vi "New Worker Name UI.vi"(11 "Starting Name":string) -> (0 "New Project?":bool, 1 "Add to Project":refnum<vi>, 2 "Cancelled?":bool, 3 "New Name":string)   [LabVIEW 2020, in "FlexBlocks.lvlib"]
uses:
  FlexBlocks.lvlib
panel:
  in  "Project":string(combo)
  in  "Add To Project":bool
  in  "Cancel":bool
  in  "OK":bool
  # "Enter the name of the new Worker to create:"
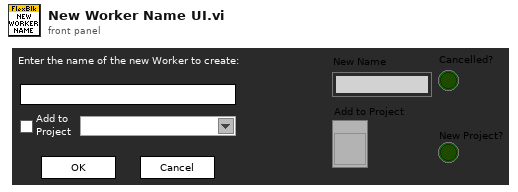
[diagram p1: front panel]
types:
  T1 = typedef "FlexBlocks.lvlib/Paths.ctl" = cluster{"FlexBlocks":path, "Workers Root":path, "Specialized Editors":path, "Worker Template":path, "Editor Template":path, "Express Template":path}
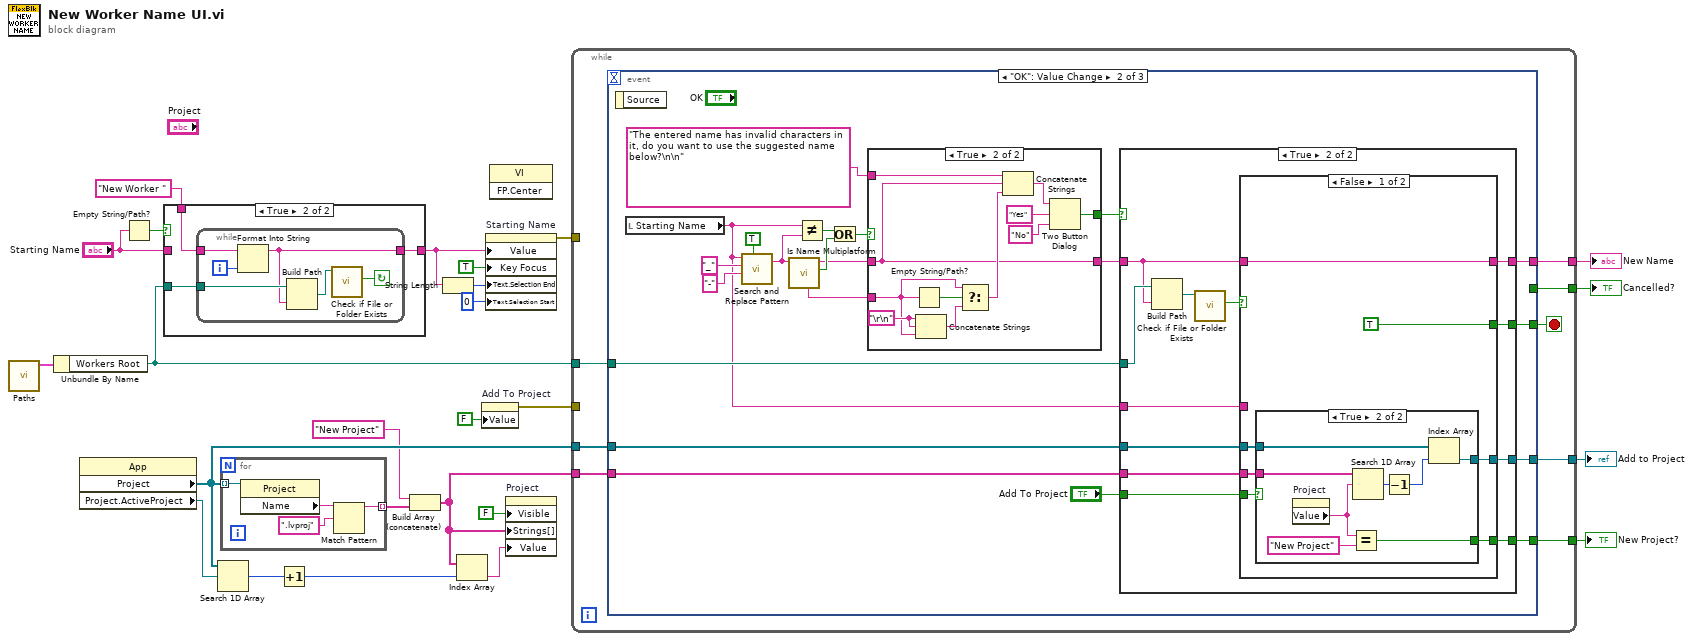
[diagram p0: block diagram]
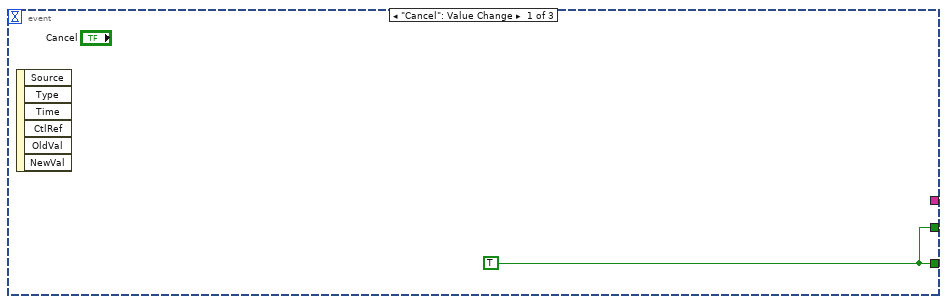
[diagram p3: hidden frame]
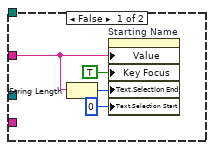
[diagram p4: hidden frame]
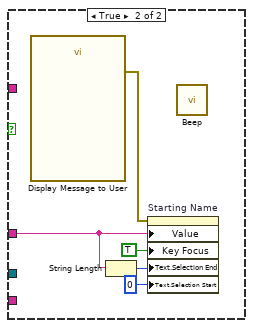
[diagram p6: hidden frame]
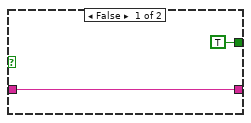
[diagram p7: hidden frame]
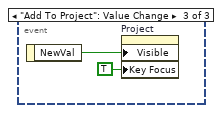
[diagram p8: hidden frame]
diagram:
  n1 = call "Paths.vi"() -> ("Paths"=w23:T1)  [unwired: 11 in]
  n2 = Unbundle By Name(w23) -> ("Workers Root"=w16:path)
  n3 = property class="App"() -> ("Project"=w8:refnum<vi>[], "Project.ActiveProject"=w12:refnum<vi>)  [unwired: 2 in, 2 out]
  n4 = Empty String/Path?(string/path="Starting Name") -> (empty?=w25:bool)
  n5 = case shown="True" w25 {
    tunnel: "Starting Name" -> [w26 _]
    tunnel: w16 -> [_ w29]
    tunnel: [w26 w28] -> w21
    tunnel: "New Worker " -> [_ w27]
    frame False {
    }
    frame True {
      n6 = while {
        tunnel: w29 -> [w34]
        tunnel: [w31] -> w28
        tunnel: w27 -> [w30]
        i -> [w35]
        stop <- w32 continue-if-true
        n7 = Format Into String(initial string=w30, w35) -> (resulting string=w31:string)  [unwired: 2 in, 1 out]
        n8 = Build Path(base path=w34, name or relative path=w31) -> (appended path=w33:path)
        n9 = call <vilib>:"Check if File or Folder Exists.vi"("path"=w33) -> ("file or folder exists?"=w32:bool)  [unwired: 8 in, 2 out]
      }
    }
  }
  n10 = Search 1D Array(1D array=w8, element=w12) -> (index of element=w11:i32)  [unwired: 1 in]
  n11 = for {
    tunnel: w8 -> [w39] mode=indexing
    tunnel: [w36] -> w9 mode=indexing
    n12 = property class="Project"(reference=w39) -> ("Name"=w38:string)  [unwired: 1 in, 2 out]
    n13 = Match Pattern(string=w38, regular expression=".lvproj") -> (before substring=w36:string)  [unwired: 1 in, 3 out]
  }
  n14 = Increment(x=w11) -> (x+1=w3:i32)
  n15 = Build Array (concatenate)("New Project", w9) -> (w5:string[])
  n16 = String Length(string=w21) -> (length=w20:i32)
  n17 = Index Array(array=w5, index=w3) -> (element=w10:string)
  n18 = property on="Add To Project" class="Bool (strict)"("Value"=FALSE ("Add To Project")) -> (error out=w1:errorcluster)  [unwired: 2 in, 1 out]
  n19 = property on="Starting Name" class="Str"("Value"=w21, "Key Focus"=TRUE, "Text.Selection End"=w20, "Text.Selection Start"=u32 0 ("Text.Selection:Start")) -> (error out=w18:errorcluster)  [unwired: 2 in, 1 out]
  n20 = invoke class="VI" method="FP.Center"() -> ()  [unwired: 3 in, 3 out]
  n21 = property on="Project" class="CmbBox"("Visible"=FALSE, "Strings[]"=w5, "Value"=w10) -> ()  [unwired: 2 in, 2 out]
  n22 = while {
    tunnel: w18 -> [_]
    tunnel: [w46] -> w17
    tunnel: w16 -> [w45]
    tunnel: [w44] -> w14
    tunnel: w5 -> [w43]
    tunnel: w8 -> [w42]
    tunnel: [w41] -> w7
    tunnel: [w40] -> w6
    tunnel: w1 -> [_]
    stop <- w47 stop-if-true
    n23 = event shown="[1] \"OK\": Value Change" {
      selector: _ -> [_ _ _]
      dyn-events: _ -> [_ _ _]
      timeout: _ -> [_ _ _]
      tunnel: [w48 w56 _] -> w47
      tunnel: [w48 _ _] -> w46
      tunnel: w45 -> [_ w57 _]
      tunnel: [_ w55 _] -> w44
      tunnel: w43 -> [_ w53 _]
      tunnel: w42 -> [_ w52 _]
      tunnel: [_ w50 _] -> w41
      tunnel: [_ w49 _] -> w40
      event "Cancel": Value Change {
        w48 = TRUE
        n24 = event-data() -> ()  [unwired: 1 in, 6 out]
      }
      event "OK": Value Change {
        n25 = event-data() -> ()  [unwired: 1 in, 1 out]
        n26 = local read "Starting Name"() -> (w54:string)
        n27 = call <vilib>:"Search and Replace Pattern.vi"("string"=w54, "regular expression (\"\")"="_" ("regular expression (\"\")"), "replace string (\"\")"="-" ("replace string (\"\")"), "replace all? (F)"=TRUE) -> ("result string"=w63:string)  [unwired: 1 in, 1 out]
        n28 = call <vilib>:"Is Name Multiplatform.vi"("filename"=w63) -> ("filename had conflict"=w68:bool, "suggested filename"=w67:string, "problem description"=w69:string)  [unwired: 6 in, 2 out]
        n29 = Not Equal?(x=w54, y=w63) -> (x != y?=w61:bool)
        n30 = Or(x=w61, y=w68) -> (x .or. y?=w62:bool)
        n31 = case shown="True" w62 {
          tunnel: w69 -> [_ w112]
          tunnel: w67 -> [w107 w108]
          tunnel: "The entered name has invalid characters in it, do you want to use the suggested name below?\n\n" -> [_ w116]
          tunnel: [TRUE ("T button?") w109] -> w59
          tunnel: [w107 w108] -> w58
          frame False {
          }
          frame True {
            w114 = "\r\n"
            n32 = Empty String/Path?(string/path=w112) -> (empty?=w115:bool)
            n33 = Concatenate Strings(w114, w114, w112) -> (w113:string)
            n34 = Select(t=w112, s=w115, f=w113) -> (s? t:f=w111:string)
            n35 = Concatenate Strings(w116, w108, w111) -> (w110:string)
            n36 = Two Button Dialog(message=w110, 1:"No" ("F button name (\"Cancel\")"), 2:"Yes" ("T button name (\"OK\")")) -> (T button?=w109:bool)
          }
        }
        n37 = case shown="True" w59 {
          tunnel: w58 -> [_ w81]
          tunnel: w57 -> [_ w85]
          tunnel: [_ w82] -> w56
          tunnel: [_ w80] -> w55
          tunnel: w54 -> [w70 w79]
          tunnel: w53 -> [_ w78]
          tunnel: w52 -> [_ w77]
          tunnel: "Add To Project" -> [_ w76]
          tunnel: [_ w75] -> w50
          tunnel: [_ w74] -> w49
          frame False {
            n38 = String Length(string=w70) -> (length=w73:i32)
            n39 = property on="Starting Name" class="Str"("Value"=w70, "Key Focus"=TRUE, "Text.Selection End"=w73, "Text.Selection Start"=u32 0 ("Text.Selection:Start")) -> ()  [unwired: 2 in, 2 out]
          }
          frame True {
            n40 = Build Path(base path=w85, name or relative path=w81) -> (appended path=w84:path)
            n41 = call <vilib>:"Check if File or Folder Exists.vi"("path"=w84) -> ("file or folder exists?"=w83:bool)  [unwired: 8 in, 2 out]
            n42 = case shown="False" w83 {
              tunnel: [TRUE _] -> w82
              tunnel: w81 -> [w91 _]
              tunnel: [w91 _] -> w80
              tunnel: w79 -> [_ w101]
              tunnel: w78 -> [w89 _]
              tunnel: w77 -> [w88 _]
              tunnel: w76 -> [w90 _]
              tunnel: [w87 _] -> w75
              tunnel: [w86 _] -> w74
              frame False {
                n43 = case shown="True" w90 {
                  tunnel: w89 -> [_ w100]
                  tunnel: w88 -> [_ w99]
                  tunnel: [_ w97] -> w87
                  tunnel: [_ w94] -> w86
                  frame False {
                  }
                  frame True {
                    n44 = property on="Project" class="CmbBox"() -> ("Value"=w96:string)  [unwired: 2 in, 2 out]
                    n45 = Equal?(x=w96, y="New Project") -> (x = y?=w94:bool)
                    n46 = Search 1D Array(1D array=w100, element=w96) -> (index of element=w98:i32)  [unwired: 1 in]
                    n47 = Decrement(x=w98) -> (x-1=w93:i32)
                    n48 = Index Array(array=w99, index=w93) -> (element=w97:refnum<vi>)
                  }
                }
              }
              frame True {
                n49 = call "Display Message to User"() -> ("error out"=w102:errorcluster)  [unwired: 10 in, 1 out]
                n50 = String Length(string=w101) -> (length=w104:i32)
                n51 = property on="Starting Name" class="Str"(error in=w102, "Value"=w101, "Key Focus"=TRUE, "Text.Selection End"=w104, "Text.Selection Start"=u32 0 ("Text.Selection:Start")) -> ()  [unwired: 1 in, 2 out]
                n52 = call <vilib>:"Beep.vi"() -> ()  [unwired: 12 in]
              }
            }
          }
        }
      }
      event "Add To Project": Value Change {
        n53 = event-data() -> ("NewVal"=w120:bool)  [unwired: 1 in]
        n54 = property on="Project" class="CmbBox"("Visible"=w120, "Key Focus"=TRUE) -> ()  [unwired: 2 in, 2 out]
      }
    }
  }
  "Cancelled?" <- w17
  "New Name" <- w14
  "Add to Project" <- w7
  "New Project?" <- w6
